vi "Launch Login.vi"(8 "error in (no error)":errorcluster, 11 "[C] User Management in":refnum<class "[C] User Management.lvclass">) -> (0 "error out":errorcluster, 3 "[C] User Management out":refnum<class "[C] User Management.lvclass">)   [LabVIEW 2020, in "[C] User Management.lvlib" / "[C] User Management.lvclass"]
uses:
  [C] User Management.lvclass
  C:/Program Files (x86)/National Instruments/LabVIEW 2020/vi.lib/ActorFramework/Actor/Actor.lvclass
  [V] Login/[V] Login/[V] Login.lvclass
  [C] User Management.lvclass/[C] User Management.ctl
  [V] Login/[V] Login/[V] Login.lvclass/[V] Login.ctl
  [V] Login/[V] Login/Accessor/Write title.vi
  [V] Login/[V] Login/Accessor/Write enable rmb user.vi
  [V] Login/[V] Login/Accessor/Write recent user list.vi
  <vilib>/ActorFramework/Actor/Actor.lvclass
  [Data] Recent User/[Data] Recent User.lvclass
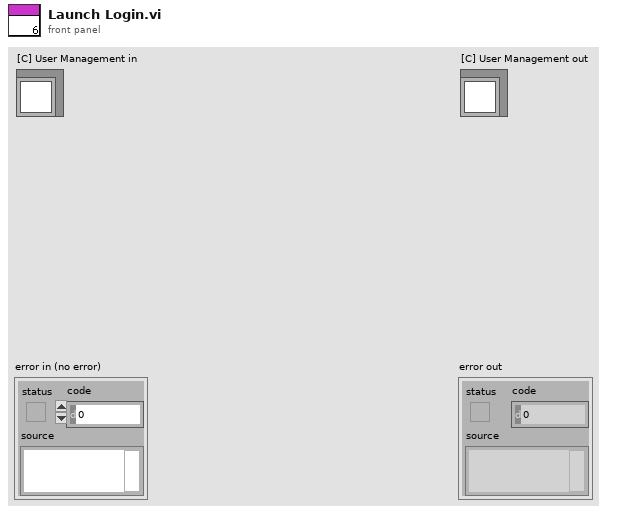
[diagram p1: front panel]
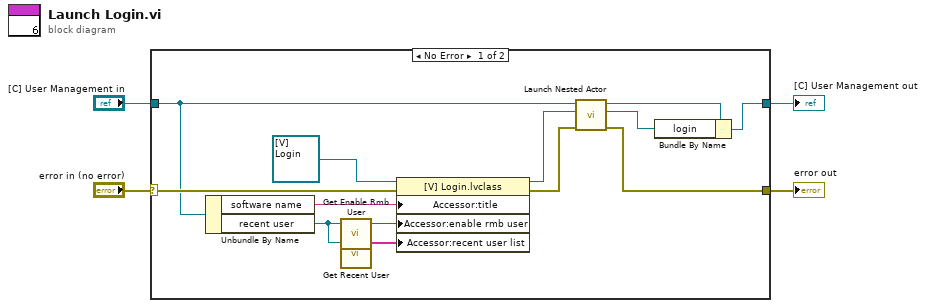
[diagram p0: block diagram]
diagram:
  n1 = case shown="No Error" "error in (no error)" {
    selector: "error in (no error)" -> [w17 w19]
    tunnel: [w13 w19] -> w3
    tunnel: [w15 w18] -> w1
    tunnel: "[C] User Management in" -> [w9 w18]
    frame No Error {
      n2 = Unbundle By Name(w9) -> ("software name"=w8:string, "recent user"=w6:refnum<class "[Data] Recent User.lvclass">)
      n3 = call "Get Enable Rmb User.vi"("[Data] Recent User in"=w6) -> ("enable rmb user"=w7:bool)  [unwired: 4 in]
      n4 = call "Get Recent User.vi"("[Data] Recent User in"=w6) -> ("recent user list"=w5:string[])  [unwired: 4 in]
      n5 = property class="[V] Login.lvclass"(reference=refnum<class "[V] Login.lvclass"> refnum ("[V] Login.lvlib:[V] Login.lvclass"), error in=w17, "Accessor:title"=w8, "Accessor:enable rmb user"=w7, "Accessor:recent user list"=w5) -> (reference out=w11:refnum<class "[V] Login.lvclass">, error out=w12:errorcluster)
      n6 = call <vilib>:"Launch Nested Actor.vi"("error in (no error)"=w12, "Nested Actor"=w11, "Caller Actor in"=w9) -> ("error out"=w13:errorcluster, "Nested Actor's Enqueuer"=w14:refnum<class "Message Enqueuer.lvclass">, "Caller Actor out"=w16:refnum<class "[C] User Management.lvclass">)  [unwired: 6 in]
      n7 = Bundle By Name(cluster=w16, "login"=w14) -> (w15:refnum<class "[C] User Management.lvclass">)
    }
    frame Error {
    }
  }
  "error out" <- w3
  "[C] User Management out" <- w1
